vi "X UserEvent Facade.vi"(0 "Data In":T4, 2 "Display State In":T2, 3 "Container State":T3) -> (6 "Data Out":T4, 7 "Display State Out":T2, 8 "Action":T1)   [LabVIEW 2009, in "XControlUserEvents.xctl"]
doc: "Demonstration of an XControl.\n\nAAL 9/09"
uses:
  XControlUserEvents.xctl
  XControl with User Events Data.ctl
  <vilib>/_xctls/Container State.ctl
  XControl with User Events State.ctl
  <vilib>/_xctls/Action.ctl
  <vilib>/_xctls/XControlSupport.lvlib
panel:
  in  "Stop":bool
  in  "Button 3":bool
  in  "Button 2":bool
  in  "Button 1":bool
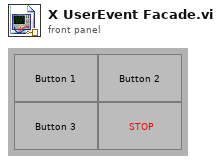
[diagram p1: front panel]
types:
  T1 = typedef "XControlSupport.lvlib/Action.ctl" = cluster{"Data Changed?":bool, "State Changed?":bool, "Action Name":string}
  T2 = typedef "XControlUserEvents.xctl/XControl with User Events State.ctl" = cluster{"Numeric":dbl, "user event":refnum<user-event>, "String":string}
  T3 = typedef "XControlSupport.lvlib/Container State.ctl" = cluster{"Indicator?":bool, "Run Mode?":bool, " Refnum":refnum<vi>}
  T4 = typedef "XControlUserEvents.xctl/XControl with User Events Data.ctl" = string
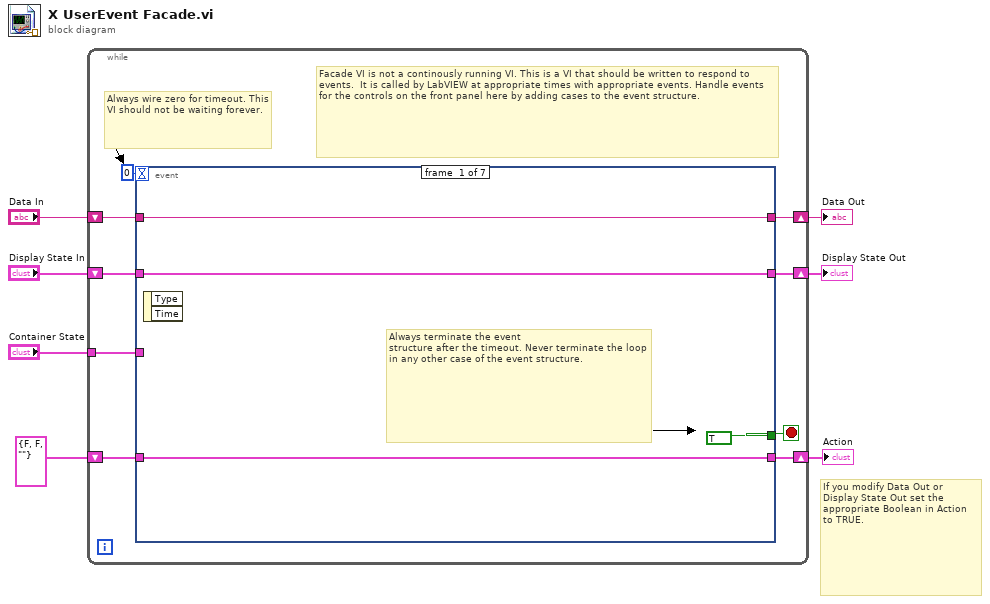
[diagram p0: block diagram]
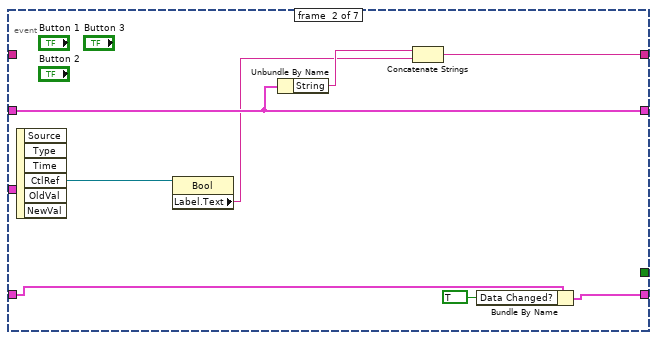
[diagram p2: hidden frame]
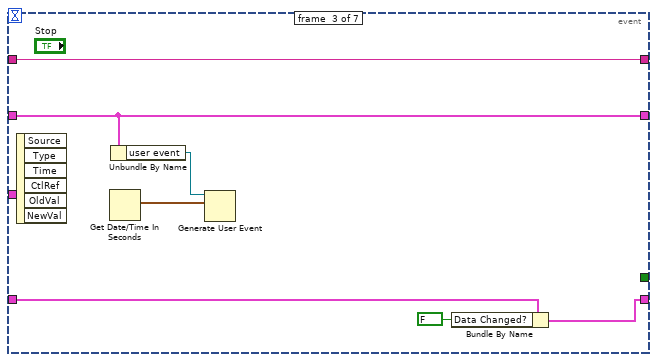
[diagram p3: hidden frame]
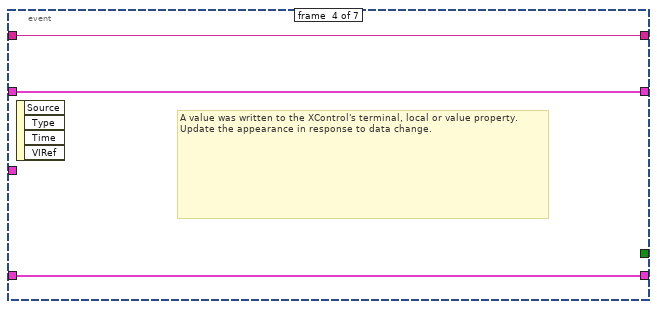
[diagram p4: hidden frame]
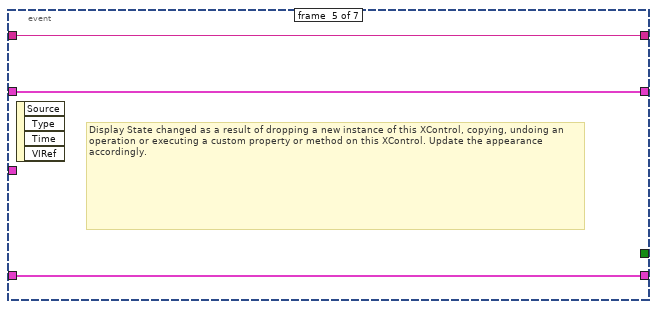
[diagram p5: hidden frame]
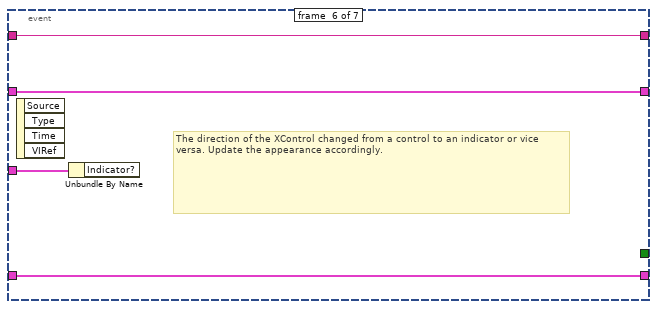
[diagram p6: hidden frame]
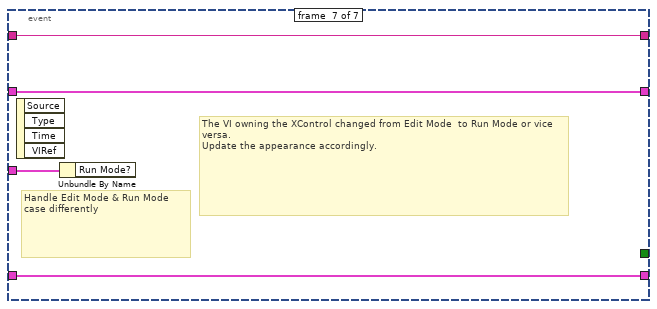
[diagram p7: hidden frame]
diagram:
  # "If you modify Data Out or\nDisplay State Out set the\nappropriate Boolean in Action\nto TRUE."
  n1 = while {
    shift-right: [w15] -> w4
    shift-left: "Display State In" -> [w16]
    tunnel: "Container State" -> [w12]
    shift-right: [w10] -> w7
    shift-left: "Data In" -> [w11]
    shift-right: [w8] -> w2
    shift-left: T1 {"Data Changed?"=FALSE, "State Changed?"=FALSE, "Action Name"=""} ("Action") -> [w9]
    stop <- w14 stop-if-true
    # "Facade VI is not a continously running VI. This is a VI that should be written to respond to events.  It is called by LabVIEW at appropriate times with appropriate events. Handle events for the controls on the front panel here by adding cases to the event structure."
    # "Always wire zero for timeout. This\nVI should not be waiting forever."
    n2 = event shown="[2] \"Stop\": Value Change" {
      selector: _ -> [_ _ _ _ _ _ _]
      dyn-events: _ -> [_ _ _ _ _ _ _]
      timeout: 0 -> [_ _ _ _ _ _ _]
      tunnel: w16 -> [w18 w24 w33 w37 w41 w44 w48]
      tunnel: [w18 w24 w33 w37 w41 w44 w48] -> w15
      tunnel: [TRUE _ _ _ _ _ _] -> w14
      tunnel: w12 -> [_ _ _ _ _ w45 w49]
      tunnel: w11 -> [w17 _ w29 w38 w40 w43 w47]
      tunnel: [w17 w21 w29 w38 w40 w43 w47] -> w10
      tunnel: [w19 w25 w31 w36 w39 w42 w46] -> w8
      tunnel: w9 -> [w19 w27 w32 w36 w39 w42 w46]
      event #0 {
        # "Always terminate the event\nstructure after the timeout. Never terminate the loop in any other case of the event structure."
        n3 = event-data() -> ()  [unwired: 1 in, 2 out]
      }
      event #1 {
        n4 = event-data() -> ("CtlRef"=w28:refnum<vi>)  [unwired: 1 in, 5 out]
        n5 = property class="Bool"(reference=w28) -> ("Label.Text"=w22:string)  [unwired: 1 in, 2 out]
        n6 = Unbundle By Name(w24) -> ("String"=w23:string)
        n7 = Concatenate Strings(w23, w22) -> (w21:string)
        n8 = Bundle By Name(cluster=w27, "Data Changed?"=TRUE) -> (w25:T1)
      }
      event #2 {
        n9 = event-data() -> ()  [unwired: 1 in, 6 out]
        n10 = Get Date/Time In Seconds() -> (seconds since 1Jan1904=w35:timestamp)
        n11 = Unbundle By Name(w33) -> ("user event"=w34:refnum<user-event>)
        n12 = Generate User Event(user event=w34, event data cluster=w35) -> ()  [unwired: 1 in, 2 out]
        n13 = Bundle By Name(cluster=w32, "Data Changed?"=FALSE) -> (w31:T1)
      }
      event #3 {
        # "A value was written to the XControl's terminal, local or value property.\nUpdate the appearance in response to data change."
        n14 = event-data() -> ()  [unwired: 1 in, 4 out]
      }
      event #4 {
        # "Display State changed as a result of dropping a new instance of this XControl, copying, undoing an operation or executing a custom property or method on this XControl. Update the appearance accordingly."
        n15 = event-data() -> ()  [unwired: 1 in, 4 out]
      }
      event #5 {
        # "The direction of the XControl changed from a control to an indicator or vice versa. Update the appearance accordingly."
        n16 = event-data() -> ()  [unwired: 1 in, 4 out]
        n17 = Unbundle By Name(w45) -> ()  [unwired: 1 out]
      }
      event #6 {
        # "The VI owning the XControl changed from Edit Mode  to Run Mode or vice versa.\nUpdate the appearance accordingly."
        # "Handle Edit Mode & Run Mode\ncase differently"
        n18 = event-data() -> ()  [unwired: 1 in, 4 out]
        n19 = Unbundle By Name(w49) -> ()  [unwired: 1 out]
      }
    }
  }
  "Display State Out" <- w4
  "Data Out" <- w7
  "Action" <- w2
